vi "Save for 2020.vi"   [LabVIEW 2023]
panel:
  # "Run me to populate the folder"
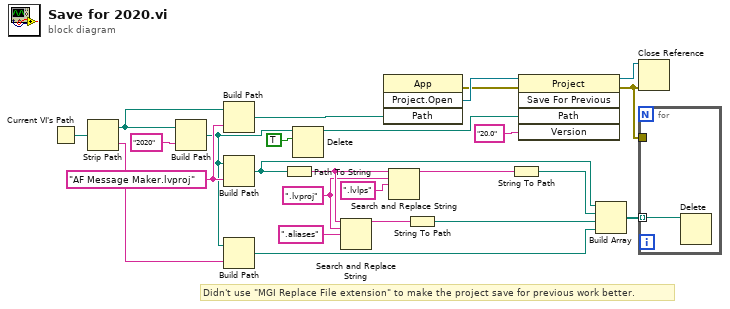
[diagram p0: block diagram]
diagram:
  w2 = ".lvproj" ("search string")
  w15 = "AF Message Maker.lvproj" ("name or relative path")
  # "Didn't use \"MGI Replace File extension\" to make the project save for previous work better."
  n1 = Current VI's Path() -> (path=w25:path)
  n2 = Strip Path(path=w25) -> (stripped path=w19:path, name=w13:string)
  n3 = Build Path(base path=w19, name or relative path="2020") -> (appended path=w14:path)
  n4 = Build Path(base path=w19, name or relative path=w15) -> (appended path=w18:path)
  n5 = Build Path(base path=w14, name or relative path=w15) -> (appended path=w8:path)
  n6 = Build Path(base path=w14, name or relative path=w13) -> (appended path=w12:path)
  n7 = Path To String(path=w8) -> (string=w5:string)
  n8 = Delete(path (use dialog)=w14, entire hierarchy (F)=TRUE) -> (deleted path=w23:path)  [unwired: 3 in, 2 out]
  n9 = Search and Replace String(input string=w5, search string=w2, replace string=".aliases" ("replace string (\"\")")) -> (result string=w4:string)  [unwired: 5 in, 3 out]
  n10 = invoke class="App" method="Project.Open"("Path"=w18) -> (error out=w16:errorcluster, "Project:Open"=w20:refnum<vi>)  [unwired: 3 in, 2 out]
  n11 = Search and Replace String(input string=w5, search string=w2, replace string=".lvlps" ("replace string (\"\")")) -> (result string=w7:string)  [unwired: 5 in, 3 out]
  n12 = String To Path(string=w4) -> (path=w3:path)
  n13 = String To Path(string=w7) -> (path=w6:path)
  n14 = invoke class="Project" method="Save For Previous"(reference=w20, error in=w16, "Path"=w23, "Version"="20.0") -> (reference out=w17:refnum<vi>, error out=w10:errorcluster)  [unwired: 1 in, 3 out]
  n15 = Build Array(w8, w6, w3, w12) -> (w11:path[])
  n16 = Close Reference(reference=w17, error in (no error)=w10) -> ()  [unwired: 1 out]
  n17 = for {
    tunnel: w11 -> [w26] mode=indexing
    tunnel: w10 -> [_]
    n18 = Delete(path (use dialog)=w26) -> ()  [unwired: 4 in, 3 out]
  }
